vi "Kalibrierung Differnzdrucksensoren.vi"(8 "Nullpunktverschiebung":sgl, 9 "Kalibrierter Wert":sgl, 11 "Normierter Wert":sgl) -> (3 "Kalibrierter Wert":sgl)   [LabVIEW 2020, in "Verwaltung - cRIO.lvlib"]
uses:
  Verwaltung - cRIO.lvlib
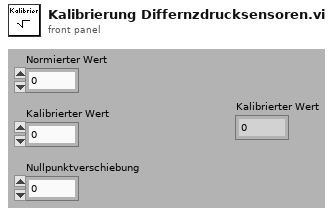
[diagram p1: front panel]
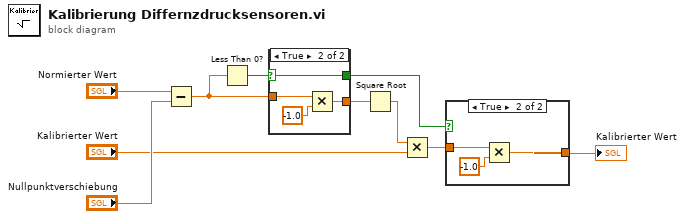
[diagram p0: block diagram]
diagram:
  n1 = Subtract(x="Normierter Wert", y="Nullpunktverschiebung") -> (x-y=w2:sgl)
  n2 = Less Than 0?(x=w2) -> (x < 0?=w9:bool)
  n3 = case shown="True" w9 {
    selector: w9 -> [w11 w13]
    tunnel: w2 -> [w12 w15]
    tunnel: [w12 w14] -> w8
    tunnel: [w11 w13] -> w4
    frame False {
    }
    frame True {
      n4 = Multiply(x=w15, y=sgl -1.0) -> (x*y=w14:sgl)
    }
  }
  n5 = Square Root(x=w8) -> (sqrt(x)=w7:sgl)
  n6 = Multiply(x=w7, y="Kalibrierter Wert") -> (x*y=w5:sgl)
  n7 = case shown="True" w4 {
    tunnel: w5 -> [w17 w19]
    tunnel: [w17 w18] -> w1
    frame False {
    }
    frame True {
      n8 = Multiply(x=w19, y=sgl -1.0) -> (x*y=w18:sgl)
    }
  }
  "Kalibrierter Wert" <- w1
